vi "usrp set rx rate.vi"(8 "error in (no error)":errorcluster, 9 "chan":u64, 10 "rate":dbl, 11 "h":u64) -> (0 "error out":errorcluster, 2 "function return":u32(ring), 3 "h 2":u64)   [LabVIEW 2023, in "uhd.lvlib"]
doc: "UHD_API uhd_error uhd_usrp_set_rx_rate(uhd_usrp_handle h, double rate, size_t chan);"
uses:
  <userlib>/uhd/uhd.lvlib
  <userlib>/uhd/uhd.dll
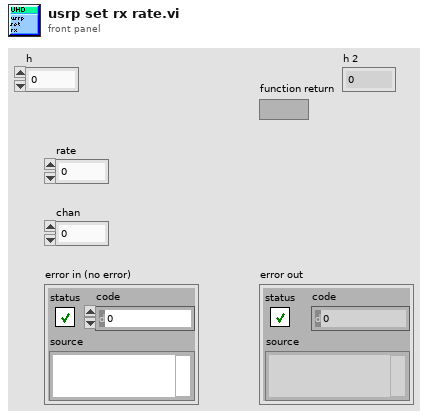
[diagram p1: front panel]
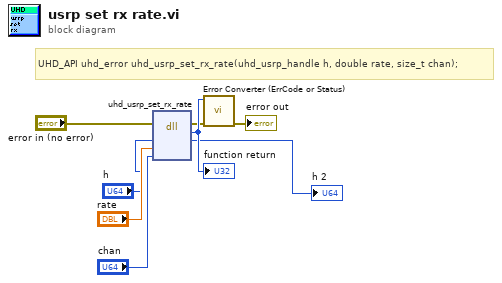
[diagram p0: block diagram]
diagram:
  # "UHD_API uhd_error uhd_usrp_set_rx_rate(uhd_usrp_handle h, double rate, size_t chan);"
  n1 = dll-call lib="C:/Program Files/National Instruments/LabVIEW 2023/user.lib/uhd/uhd.dll" fn="uhd_usrp_set_rx_rate"(error in="error in (no error)", "h"="h", "rate"="rate", "chan"="chan") -> (error out=w4:errorcluster, "return type"=w8:u32, "h"=→"h 2":u64)  [unwired: 4 in, 1 out]
  "function return" <- w8
  n2 = call <userlib>:"Error Converter (ErrCode or Status).vi"("error in (no error)"=w4, "error code"=w8) -> ("error out"=→"error out":errorcluster)  [unwired: 9 in]
